vi "CloseServer.vi"(3 "Server":string) -> (0 "Active Servers Out":string[][](array[string]))   [LabVIEW 2013]
uses:
  _ROSDefinition.vi
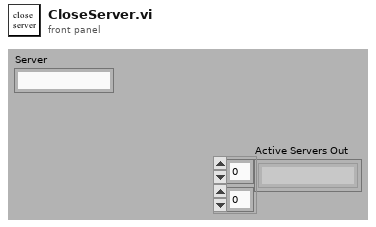
[diagram p1: front panel]
types:
  T1 = cluster{"server vi":string, "reference":refnum<vi>, "Description":string[], "Connected":bool}[]
  T2 = cluster{"server vi":string, "reference":refnum<vi>, "Description":string[], "Connected":bool}
  T3 = enum32{"Bad", "Idle", "Run top level", "Running"}
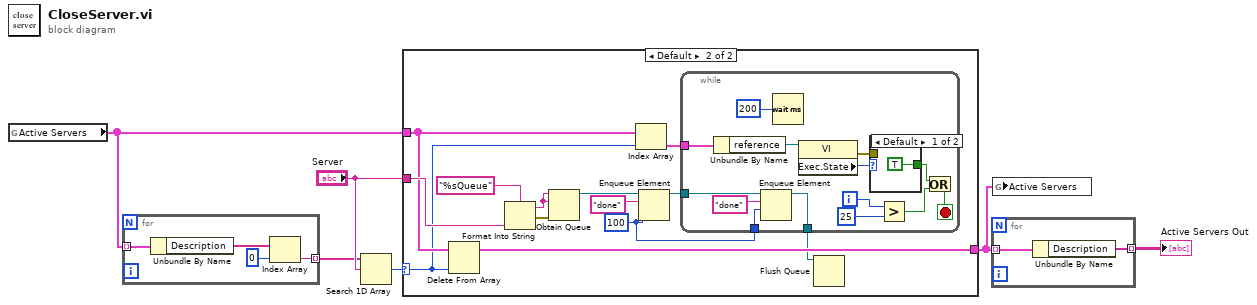
[diagram p0: block diagram]
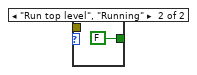
[diagram p3: hidden frame]
diagram:
  n1 = global read "_ROSDefinition.vi" "Active Servers"() -> (w3:T1)
  n2 = for {
    tunnel: [w10] -> w4 mode=indexing
    tunnel: w3 -> [w9] mode=indexing
    n3 = Unbundle By Name(w9) -> ("Description"=w7:string[])
    n4 = Index Array(array=w7, index=0 ("disabled index (col)")) -> (element=w10:string)
  }
  n5 = Search 1D Array(1D array=w4, element="Server") -> (index of element=w5:i32)  [unwired: 1 in]
  n6 = case shown="Default" w5 {
    selector: w5 -> [_ w16]
    tunnel: [w11 w18] -> w2
    tunnel: w3 -> [w11 w17]
    tunnel: "Server" -> [_ w24]
    frame -1 {
    }
    frame Default {
      w12 = 100 ("timeout in ms (-1)")
      n7 = Delete From Array(array=w17, index=w16) -> (array with subset deleted=w18:T1)  [unwired: 1 in, 1 out]
      n8 = Format Into String(format string="%sQueue" ("name (unnamed)"), w24) -> (resulting string=w20:string, error out=w19:errorcluster)  [unwired: 2 in]
      n9 = Obtain Queue(name (unnamed)=w20, element data type=w20, error in (no error)=w19) -> (queue out=w21:refnum<queue>)  [unwired: 2 in, 2 out]
      n10 = Index Array(array=w17, index=w16) -> (element=w15:T2)
      n11 = Enqueue Element(queue=w21, element="done", timeout in ms (-1)=w12) -> (queue out=w14:refnum<queue>)  [unwired: 1 in, 2 out]
      n12 = while {
        tunnel: w15 -> [w38]
        tunnel: w14 -> [w34]
        tunnel: [w32] -> w13
        tunnel: w12 -> [w25]
        i -> [w30]
        stop <- w26 stop-if-true
        n13 = Unbundle By Name(w38) -> ("reference"=w37:refnum<vi>)
        n14 = Enqueue Element(queue=w34, element="done", timeout in ms (-1)=w25) -> (queue out=w32:refnum<queue>)  [unwired: 1 in, 2 out]
        n15 = Wait (ms)(milliseconds to wait=u32 200) -> ()  [unwired: 1 out]
        n16 = property class="VI"(reference=w37) -> (error out=w31:errorcluster, "Exec.State"=w36:T3)  [unwired: 1 in, 1 out]
        n17 = case shown="Default" w36 {
          tunnel: [TRUE FALSE] -> w28
          tunnel: w31 -> [_ _]
          frame Default {
          }
          frame "Run top level", "Running" {
          }
        }
        n18 = Greater?(x=w30, y=25) -> (0:w27:bool)
        n19 = Or(x=w28, y=w27) -> (x .or. y?=w26:bool)
      }
      n20 = Flush Queue(queue=w13) -> ()  [unwired: 1 in, 3 out]
    }
  }
  n21 = for {
    tunnel: w2 -> [w42] mode=indexing
    tunnel: [w41] -> w1 mode=indexing
    n22 = Unbundle By Name(w42) -> ("Description"=w41:string[])
  }
  "Active Servers Out" <- w1
  n23 = global write "_ROSDefinition.vi" "Active Servers"(w2) -> ()
